vi "ELVIS III Check AI IRQ (in 1 sample).vi"(5 "Hysteresis":fxp<+/-,26,5>, 7 "Timed Out?":bool, 8 "Threshold":fxp<+/-,26,5>, 9 "Analog Value":fxp<+/-,26,5>, 10 "Rising Edge?":bool, 11 "Enable Interrupt?":bool) -> (3 "Interrupt Ready?":bool)   [LabVIEW 2019]
doc: "This VI checks if the analog input interrupt is triggered under the specified condition.\n<b>IRQ Number</b> specifies the identifier of the interrupt. <b>IRQ Number</b> ranges from 1 to 8 on FPGA and is shared between analog, digital, and button interrupts."
uses:
  <vilib>/Platform/TimedLoop/XDataNode/timing_clust.ctl
  <vilib>/Platform/TimedLoop/XDataNode/nitl_modes.ctl
  <vilib>/Platform/TimedLoop/XDataNode/wakeup.ctl
  <vilib>/rvi/Emulation/niFpgaSctlEmulationGetInTimedLoop.vi
  <vilib>/rvi/Emulation/niFpgaEmulationReportErrorSimple.vi
  <vilib>/rvi/Emulation/niFpgaGetClockAttributes.vi
  <vilib>/rvi/Emulation/niFpgaCriticalErrorInLSC.vi
  <vilib>/Platform/TimedLoop/XDataNode/XDataNode.xnode
  <vilib>/Platform/TimedLoop/XDataNode/XDNodeRunTimeDep.lvlib
panel:
  # "This VI checks if the analog input interrupt is triggered under the specified condition.\nIRQ Number specifies the identifier of the interrupt."
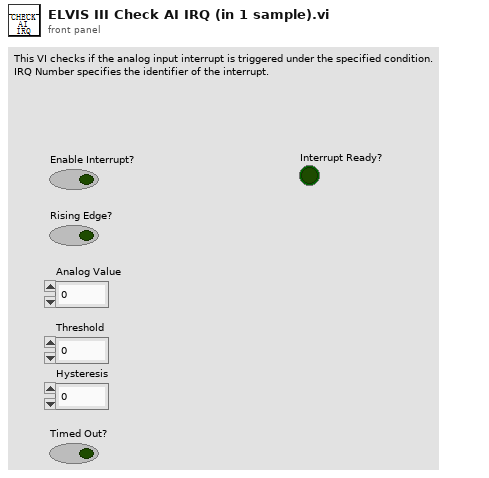
[diagram p1: front panel]
types:
  T1 = typedef "XDNodeRunTimeDep.lvlib/timing_clust.ctl" = cluster{"Expected End [f-1]":u64, "Actual End [f-1]":u64, "Finished Late? [f-1]":bool, "Expected End [i-1]":u64, "Actual End [i-1]":u64, "Finished Late? [i-1]":bool, "Expected Start [i]":u64, "Actual Start [i]":u64, "Expected Start [f]":u64, "Actual Start [f]":u64, "Source Name":string, "Structure Name":string, "Period":i64, "Deadline":i64, "Offset":i64, "Start":i64, "Priority":i32, "Timeout":i32, "Mode":T2, "Wakeup Reason":T3, "Error":errorcluster, "Source Type":string, "Secondary Source Type":string, "Global End Time":u64, "Global Start Time":u64, "Frame Duration":u64, "Iteration Duration":u64, "Assigned CPU":i32, "I/O Scan Engine Mode":u32}
  T2 = typedef "XDNodeRunTimeDep.lvlib/nitl_modes.ctl" = enum32{"No Change", "Process missed periods, maintain original phase", "Discard missed periods, maintain original phase", "Process missed periods, ignore original phase", "Discard missed periods, ignore original phase"}
  T3 = typedef "XDNodeRunTimeDep.lvlib/wakeup.ctl" = enum32{"Normal", "Aborted", "Asynchronous wakeup", "Timing source error", "Timed loop error", "Timeout"}
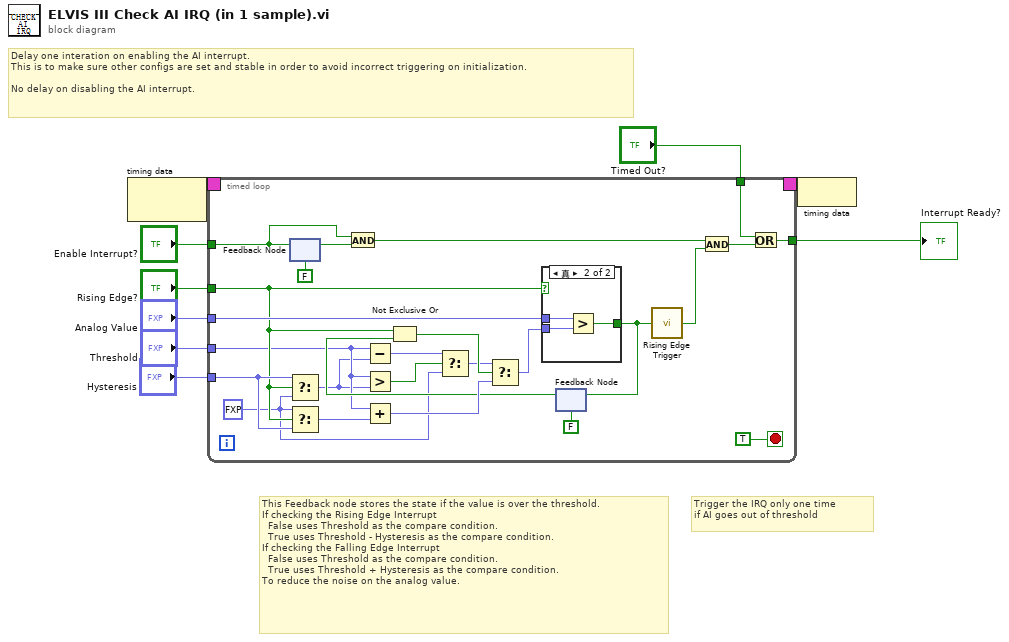
[diagram p0: block diagram]
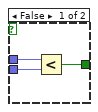
[diagram p2: hidden frame]
diagram:
  # "Delay one interation on enabling the AI interrupt.\nThis is to make sure other configs are set and stable in order to avoid incorrect triggering on initialization.\n\nNo delay on disabling the AI interrupt."
  # "Trigger the IRQ only one time \nif AI goes out of threshold"
  # "This Feedback node stores the state if the value is over the threshold.\nIf checking the Rising Edge Interrupt\n  False uses Threshold as the compare condition.\n  True uses Threshold - Hysteresis as the compare condition.\nIf checking the Falling Edge Interrupt\n  False uses Threshold as the compare condition.\n  True uses Threshold + Hysteresis as the compare condition.\nTo reduce the noise on the analog value."
  n1 = node-c288() -> (w5:T1)  [unwired: 1 in]
  n2 = timed-loop {
    timing: w5 -> [_]
    timing-out: [_] -> w4
    tunnel: "Analog Value" -> [w34]
    tunnel: "Threshold" -> [w21]
    tunnel: "Hysteresis" -> [w24]
    tunnel: "Rising Edge?" -> [w23]
    tunnel: [w26] -> w3
    tunnel: "Timed Out?" -> [w25]
    tunnel: "Enable Interrupt?" -> [w13]
    stop <- TRUE stop-if-true
    w16 = fxp<+/-,26,5> 0.0 ("f")
    n3 = feedback-in #1(w13) -> ()
    n4 = feedback #1(FALSE ("Enable Interrupt?")) -> (w12:bool)
    n5 = Select(t=w24, s=w23, f=w16) -> (s? t:f=w20:fxp<+/-,26,5>)
    n6 = Select(t=w16, s=w23, f=w24) -> (s? t:f=w22:fxp<+/-,26,5>)
    n7 = And(x=w13, y=w12) -> (x .and. y?=w11:bool)
    n8 = Subtract(x=w21, y=w20) -> (x-y=w18:fxp<+/-,27,6>)
    n9 = Greater?(x=w21, y=w20) -> (0:w19:bool)
    n10 = Add(x=w21, y=w22) -> (x+y=w32:fxp<+/-,27,6>)
    n11 = Select(t=w18, s=w19, f=w16) -> (s? t:f=w17:fxp<+/-,27,6>)
    n12 = feedback #2(FALSE ("Timed Out?")) -> (w29:bool)
    n13 = Not Exclusive Or(1:w29, 2:w23) -> (0:w28:bool)
    n14 = Select(t=w17, s=w28, f=w32) -> (s? t:f=w31:fxp<+/-,27,6>)
    n15 = case shown="真" w23 {
      tunnel: w34 -> [w37 w40]
      tunnel: w31 -> [w36 w39]
      tunnel: [w35 w38] -> w30
      frame False {
        n16 = Less?(x=w37, y=w36) -> (x < y?=w35:bool)
      }
      frame True {
        n17 = Greater?(x=w40, y=w39) -> (0:w38:bool)
      }
    }
    n18 = feedback-in #2(w30) -> ()
    n19 = call "Rising Edge Trigger.vi"("Signal"=w30) -> ("Trigger?"=w15:bool)
    n20 = And(x=w11, y=w15) -> (x .and. y?=w14:bool)
    n21 = Or(x=w25, y=w14) -> (x .or. y?=w26:bool)
  }
  "Interrupt Ready?" <- w3
  n22 = node-c288(w4) -> ()
